vi "Main.vi"(8 "error in":errorcluster, 11 "Query Data in":refnum<class "Query Data.lvclass">) -> (0 "error out":errorcluster, 3 "Query Data out":refnum<class "Query Data.lvclass">)   [LabVIEW 2018, in "Query Data.lvclass"]
doc: "The Queued Message Handler of a Worker."
uses:
  Query Data.lvclass
  D:/Program Files (x86)/National Instruments/LabVIEW 2018/vi.lib/addons/_Workers/Library/Classes/Worker/Worker.lvclass
  Initialization Data.ctl
  Query Data.lvclass/Query Data.ctl
  <vilib>/drjdpowell/SQLite Library/SQL Connection/Open (path).vi
  <vilib>/drjdpowell/SQLite Library/SQL Connection/Open (string).vi
  <vilib>/AdvancedString/Path To Command Line String.vi
  <vilib>/drjdpowell/SQLite Library/SQL Connection/Execute SQL.vi
  <vilib>/addons/_Workers/Library/Classes/Message/Enqueue Message to Self v2.vi
  <vilib>/drjdpowell/SQLite Library/SQL Connection/Connection.lvclass
  <vilib>/addons/_Workers/Library/Classes/Worker/Worker.lvclass
  <vilib>/addons/_Workers/Library/Classes/Message/Message.lvclass
  <vilib>/drjdpowell/SQLite Library/SQLite.lvlib
  D:/Program Files (x86)/National Instruments/LabVIEW 2018/vi.lib/addons/_Workers/Library/Classes/Workers Object/Workers Object.lvclass
panel:
  in  "Query Button":bool
  in  "EndTime":timestamp caption="EndTime:"
  in  "StartTime":timestamp caption="StartTime:"
  in  "Slot":T1(ring) caption="Slot:"
  in  "Results":i32(listbox)
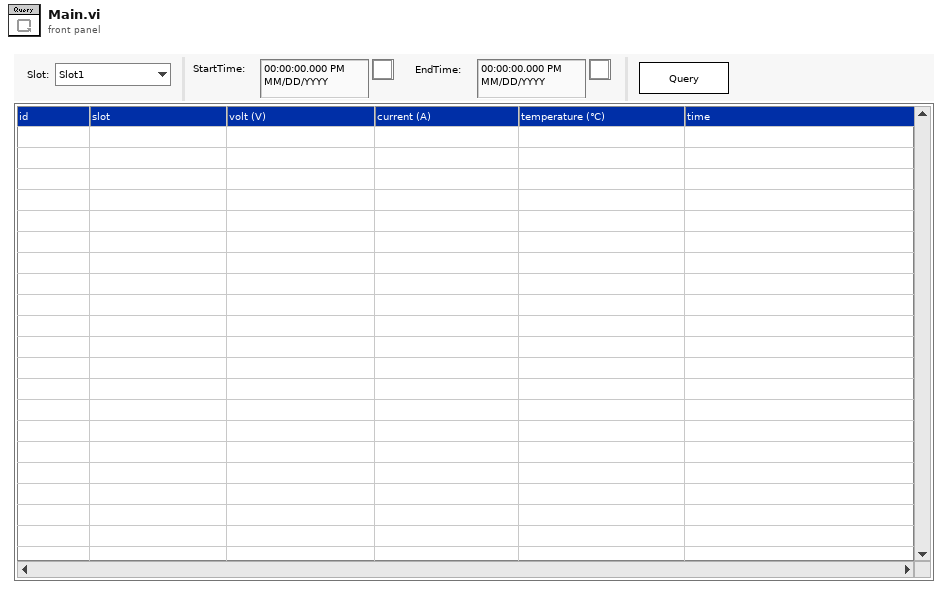
[diagram p1: front panel]
types:
  T1 = enum16{"Slot1", "Slot2", "Slot3", "Slot4", "Slot5", "Slot6", "Slot7", "Slot8", "Slot9", "Slot10"}
  T2 = typedef "Query Data.lvclass/Initialization Data.ctl" = cluster{"MainPanel":refnum<vi>}
  T3 = typedef "Workers.lvlib/Case Label.ctl" = string
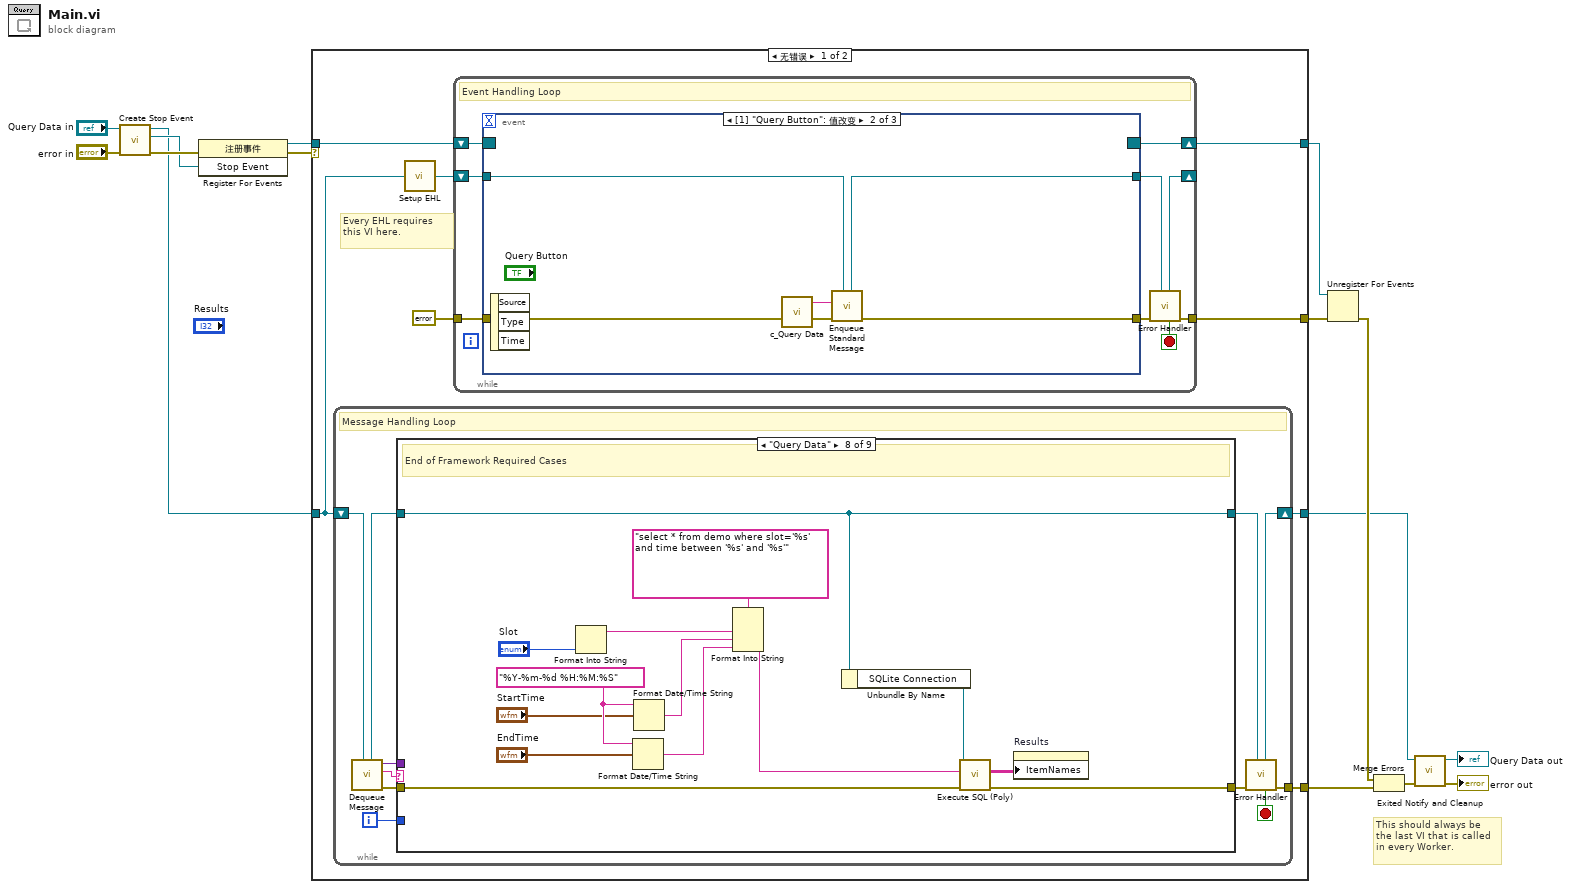
[diagram p0: block diagram]
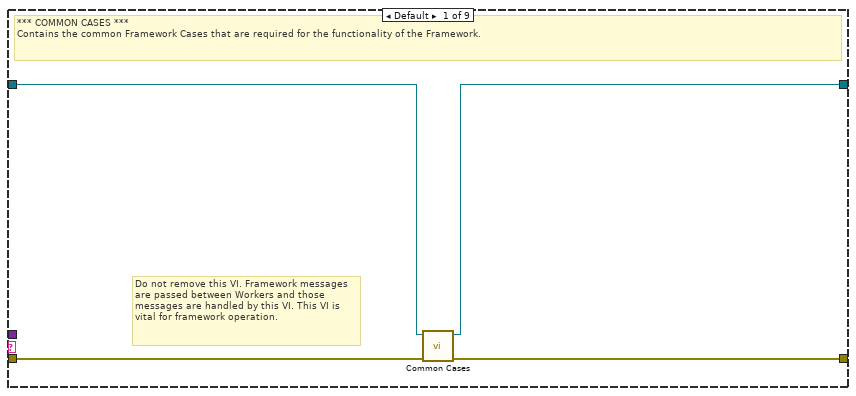
[diagram p2: hidden frame]
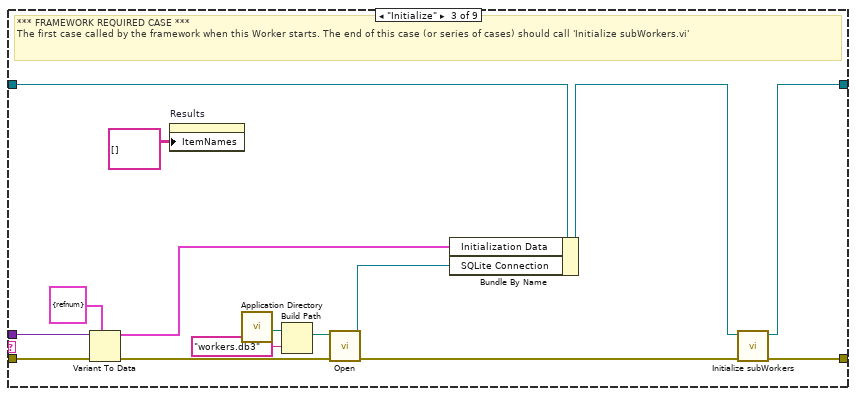
[diagram p4: hidden frame]
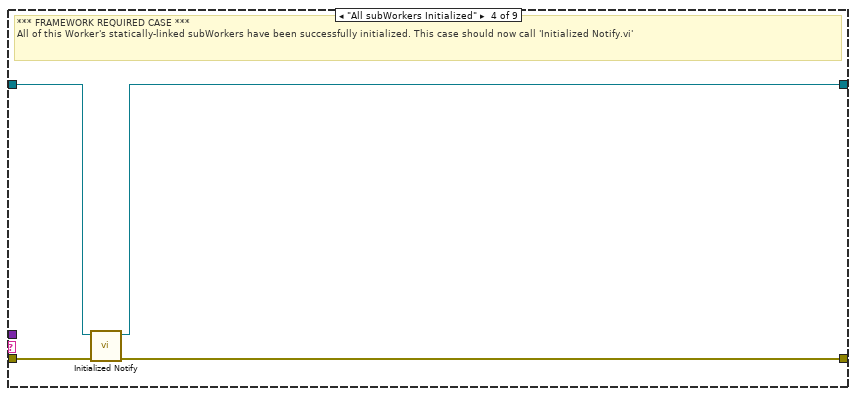
[diagram p5: hidden frame]
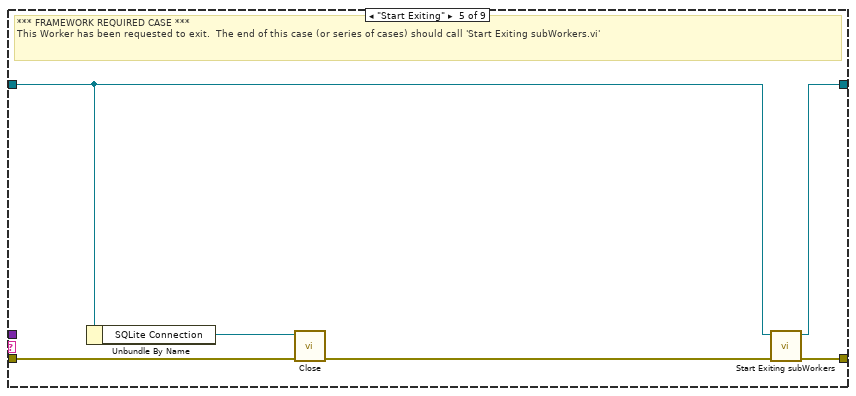
[diagram p6: hidden frame]
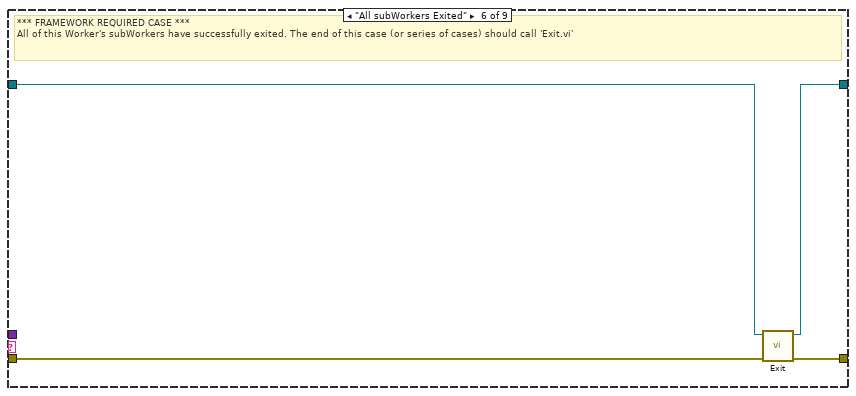
[diagram p7: hidden frame]
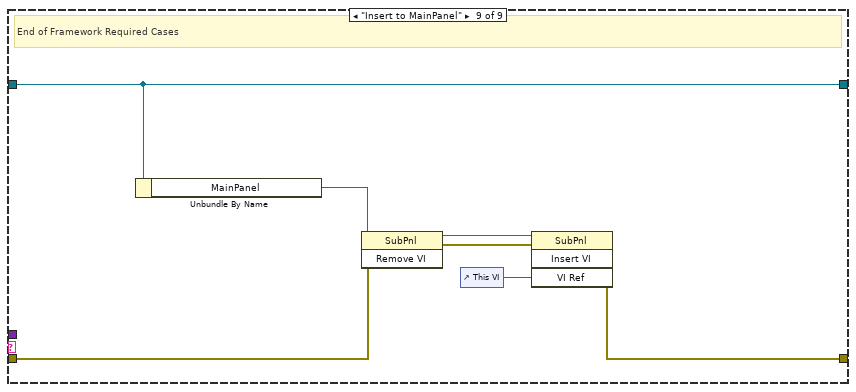
[diagram p9: hidden frame]
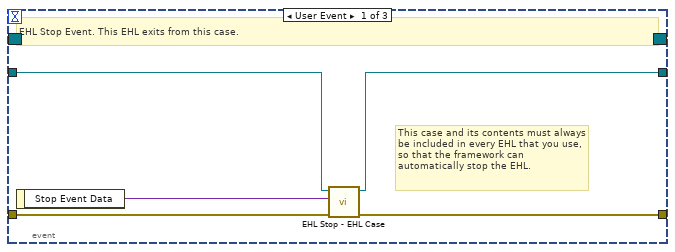
[diagram p10: hidden frame]
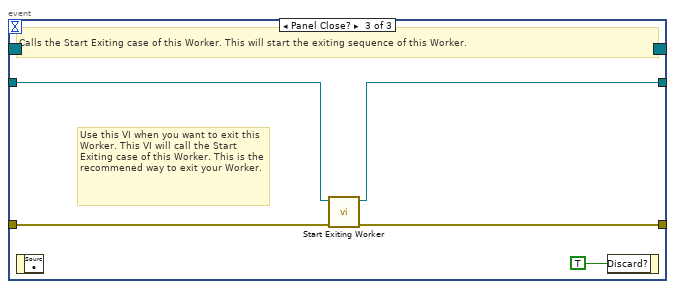
[diagram p11: hidden frame]
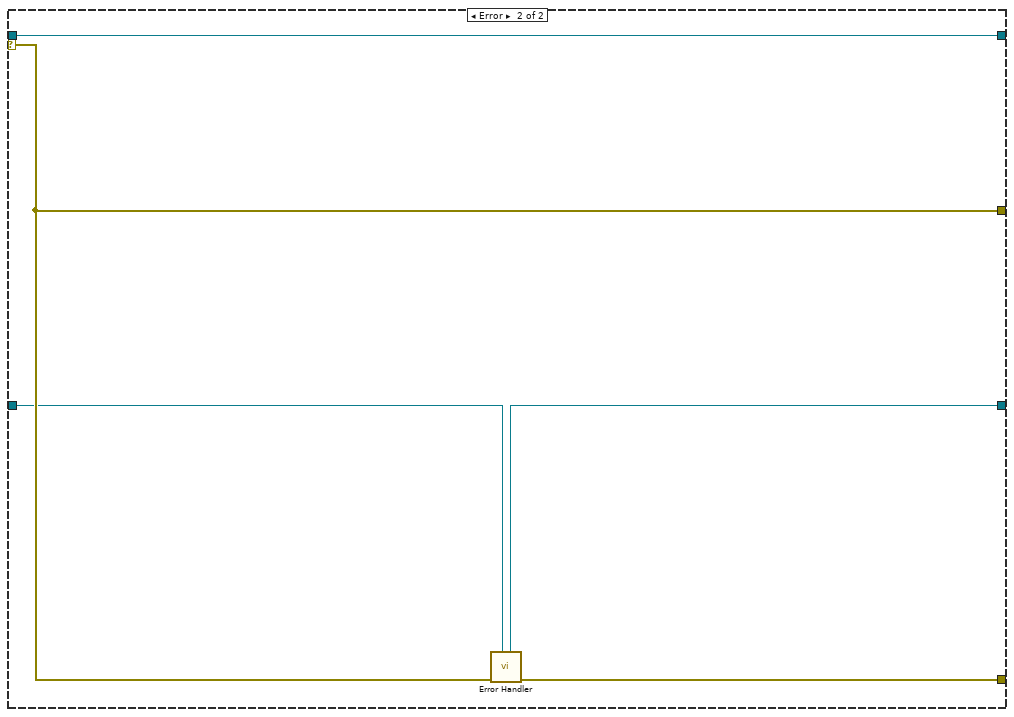
[diagram p12: hidden frame]
diagram:
  # "This should always be the last VI that is called in every Worker."
  n1 = call-dynamic "Create Stop Event.vi"("error in"="error in", "Worker"="Query Data in") -> ("error out"=w10:errorcluster, "Stop Event"=w7:refnum<user-event>, "Worker out"=w4:refnum<class "Query Data.lvclass">)  [unwired: 7 in]
  n2 = register-events(error in=w10, w7) -> (reference out=w9:refnum<event-registration>, error out=w1:errorcluster)  [unwired: 1 in]
  n3 = case shown="无错误" w1 {
    tunnel: w4 -> [w18 w118]
    tunnel: [w16 w119] -> w8
    tunnel: w9 -> [w23 w120]
    tunnel: [w20 w121] -> w14
    tunnel: [w22 w120] -> w13
    tunnel: [w17 w117] -> w11
    selector: w1 -> [_ w121]
    frame No Error {
      # "Every EHL requires\nthis VI here."
      n4 = while {
        shift-right: [w32] -> w17
        shift-left: w18 -> [w34]
        tunnel: [w33] -> w16
        i -> [w24]
        stop <- w25 stop-if-true
        # "Message Handling Loop"
        n5 = call-dynamic "Dequeue Message.vi"("Worker"=w34) -> ("error out"=w31:errorcluster, "Case out"=w26:string, "Data out"=w27:variant, "Worker out"=w29:refnum<class "Query Data.lvclass">)  [unwired: 6 in, 1 out]
        n6 = case "Worker MHL Case Structure (DO NOT CHANGE LABEL NAME)" shown="\"Query Data\"" w26 {
          tunnel: w31 -> [w38 w39 w53 w57 w62 w69 w70 w84 w87]
          tunnel: [w37 w39 w55 w56 w65 w68 w70 w83 w86] -> w30
          tunnel: w29 -> [w36 w40 w52 w59 w63 w67 w71 w85 w88]
          tunnel: [w35 w40 w54 w58 w64 w66 w71 w85 w88] -> w28
          tunnel: w27 -> [_ _ w51 _ _ _ _ _ _]
          tunnel: w24 -> [_ _ _ _ _ _ _ _ _]
          frame Default {
            # "Do not remove this VI. Framework messages are passed between Workers and those messages are handled by this VI. This VI is vital for framework operation."
            # "*** COMMON CASES ***\nContains the common Framework Cases that are required for the functionality of the Framework."
            n7 = call-dynamic "Common Cases.vi"("error in"=w38, "Worker in"=w36) -> ("error out"=w37:errorcluster, "Worker out"=w35:refnum<class "Query Data.lvclass">)  [unwired: 8 in]
          }
          frame "------ FRAMEWORK REQUIRED CASES ------" {
            # "Start of Framework Required Cases"
          }
          frame "Initialize" {
            # "*** FRAMEWORK REQUIRED CASE ***\nThe first case called by the framework when this Worker starts. The end of this case (or series of cases) should call 'Initialize subWorkers.vi'"
            n8 = Variant To Data(error in=w53, type=T2 {"MainPanel"=refnum} ("Initialization Data"), Variant=w51) -> (data=w48:T2, error out=w47:errorcluster)
            n9 = property on="Results" class="MCListbox (严格)"("ItemNames"=string[][] [] ("Item Names")) -> ()  [unwired: 2 in, 2 out]
            n10 = call <vilib>:"Application Directory.vi"() -> ("Application Directory"=w46:path)
            n11 = Build Path(base path=w46, name or relative path="workers.db3") -> (appended path=w44:path)
            n12 = call-poly <vilib>:"Open.vi"("error in (no error)"=w47, "db file"=w44) -> ("error out"=w42:errorcluster, "SQLite Connection"=w43:refnum<class "Connection.lvclass">)  [unwired: 8 in]
            n13 = Bundle By Name(cluster=w52, "Initialization Data"=w48, "SQLite Connection"=w43) -> (w49:refnum<class "Query Data.lvclass">)
            n14 = call-dynamic "Initialize subWorkers.vi"("error in"=w42, "Worker"=w49) -> ("error out"=w55:errorcluster, "dup Worker out"=w54:refnum<class "Query Data.lvclass">)  [unwired: 8 in]
          }
          frame "All subWorkers Initialized" {
            # "*** FRAMEWORK REQUIRED CASE ***\nAll of this Worker's statically-linked subWorkers have been successfully initialized. This case should now call 'Initialized Notify.vi'"
            n15 = call-dynamic "Initialized Notify.vi"("error in"=w57, "Worker"=w59) -> ("error out"=w56:errorcluster, "dup Worker out"=w58:refnum<class "Query Data.lvclass">)  [unwired: 8 in]
          }
          frame "Start Exiting" {
            # "*** FRAMEWORK REQUIRED CASE ***\nThis Worker has been requested to exit.  The end of this case (or series of cases) should call 'Start Exiting subWorkers.vi'"
            n16 = Unbundle By Name(w63) -> ("SQLite Connection"=w60:refnum<class "Connection.lvclass">)
            n17 = call-dynamic "Close.vi"("error in (no error)"=w62, "SQLite Connection in"=w60) -> ("error out"=w61:errorcluster)  [unwired: 9 in]
            n18 = call-dynamic "Start Exiting subWorkers.vi"("error_in"=w61, "Worker"=w63) -> ("error out"=w65:errorcluster, "dup Worker out"=w64:refnum<class "Query Data.lvclass">)  [unwired: 8 in]
          }
          frame "All subWorkers Exited" {
            # "*** FRAMEWORK REQUIRED CASE ***\nAll of this Worker's subWorkers have successfully exited. The end of this case (or series of cases) should call 'Exit.vi'"
            n19 = call-dynamic "Exit.vi"("error_in"=w69, "Worker"=w67) -> ("error out"=w68:errorcluster, "dup Worker out"=w66:refnum<class "Query Data.lvclass">)  [unwired: 8 in]
          }
          frame "-----------------------------------------------" {
            # "End of Framework Required Cases"
          }
          frame "Query Data" {
            w80 = "%Y-%m-%d %H:%M:%S" ("time format string (%c)")
            # "End of Framework Required Cases"
            n20 = Format Into String("Slot") -> (resulting string=w76:string)  [unwired: 3 in, 1 out]
            n21 = Format Date/Time String(time format string (%c)=w80, seconds (now)="EndTime") -> (date/time string=w74:string)  [unwired: 1 in]
            n22 = Format Date/Time String(time format string (%c)=w80, seconds (now)="StartTime") -> (date/time string=w75:string)  [unwired: 1 in]
            n23 = Format Into String(format string="select * from demo where slot='%s' and time between '%s' and '%s'", w76, w75, w74) -> (resulting string=w73:string)  [unwired: 2 in, 1 out]
            n24 = Unbundle By Name(w85) -> ("SQLite Connection"=w82:refnum<class "Connection.lvclass">)
            n25 = call-poly <vilib>:"Execute SQL (Poly).vi"("error in (no error)"=w84, "SQL"=w73, "SQLite Connection in"=w82) -> ("error out"=w83:errorcluster, "Result Set"=w72:string[][])  [unwired: 5 in, 2 out]
            n26 = property on="Results" class="MCListbox (严格)"("ItemNames"=w72) -> ()  [unwired: 2 in, 2 out]
          }
          frame "Insert to MainPanel" {
            # "End of Framework Required Cases"
            n27 = Unbundle By Name(w88) -> ("MainPanel"=w92:refnum<vi>)
            n28 = invoke class="SubPnl" method="Remove VI"(reference=w92, error in=w87) -> (reference out=w91:refnum<vi>, error out=w90:errorcluster)  [unwired: 1 in, 1 out]
            n29 = control-ref of="This VI"() -> (w89:refnum<vi>)
            n30 = invoke class="SubPnl" method="Insert VI"(reference=w91, error in=w90, "VI Ref"=w89) -> (error out=w86:errorcluster)  [unwired: 1 in, 3 out]
          }
        }
        n31 = call-dynamic "Error Handler.vi"("Worker"=w28, "error_in"=w30) -> ("error out"=w33:errorcluster, "Stop Loop"=w25:bool, "Worker out"=w32:refnum<class "Query Data.lvclass">)  [unwired: 7 in]
      }
      n32 = call-dynamic "Setup EHL.vi"("Worker"=w18) -> ("Worker out"=w19:refnum<class "Query Data.lvclass">)  [unwired: 14 in]
      n33 = while "Event Handling Loop" {
        shift-right: [w101] -> w22
        shift-left: w23 -> [w100]
        tunnel: [w96] -> w20
        tunnel: errorcluster {"status"=FALSE, "code"=0, "source"=""} ("error constant") -> [w98]
        shift-right: [w94] -> _
        shift-left: w19 -> [w99]
        stop <- w93 stop-if-true
        # "Event Handling Loop"
        n34 = event shown="[1] \"Query Button\": 值改变" {
          selector: w100 -> [_ _ _]
          dyn-events: [_ _ _] -> w101
          timeout: _ -> [_ _ _]
          tunnel: [w105 w110 w115] -> w97
          tunnel: w98 -> [w106 w111 w114]
          tunnel: w99 -> [w104 w109 w113]
          tunnel: [w103 w108 w112] -> w95
          event User Event {
            # "This case and its contents must always be included in every EHL that you use, so that the framework can automatically stop the EHL."
            # "EHL Stop Event. This EHL exits from this case."
            n35 = event-data() -> ("Stop Event Data"=w102:variant)  [unwired: 1 in]
            n36 = call <vilib>:"EHL Stop - EHL Case.vi"("error in"=w106, "Stop Event Data"=w102, "Worker"=w104) -> ("error out"=w105:errorcluster, "Worker out"=w103:refnum<class "Query Data.lvclass">)  [unwired: 7 in]
          }
          event "Query Button": Value Change {
            n37 = event-data() -> ()  [unwired: 1 in, 3 out]
            n38 = call "c_Query Data.vi"() -> ("Case Label"=w107:T3)  [unwired: 1 in]
            n39 = call-poly <vilib>:"Enqueue Standard Message.vi"("Worker"=w109, "error in"=w111, "Case Label"=w107) -> ("error out"=w110:errorcluster, "dup Worker out"=w108:refnum<class "Query Data.lvclass">)  [unwired: 7 in]
          }
          event Panel Close? {
            # "Use this VI when you want to exit this Worker. This VI will call the Start Exiting case of this Worker. This is the recommened way to exit your Worker."
            # "Calls the Start Exiting case of this Worker. This will start the exiting sequence of this Worker."
            n40 = event-data() -> ()  [unwired: 1 in, 1 out]
            n41 = call-dynamic "Start Exiting Worker.vi"("error in"=w114, "Worker"=w113) -> ("error out"=w115:errorcluster, "dup Worker out"=w112:refnum<class "Query Data.lvclass">)  [unwired: 8 in]
            n42 = event-data("Discard?"=TRUE) -> ()  [unwired: 1 in, 1 out]
          }
        }
        n43 = call-dynamic "Error Handler.vi"("Worker"=w95, "error_in"=w97) -> ("error out"=w96:errorcluster, "Stop Loop"=w93:bool, "Worker out"=w94:refnum<class "Query Data.lvclass">)  [unwired: 7 in]
      }
    }
    frame Error {
      n44 = call-dynamic "Error Handler.vi"("Worker"=w118, "error_in"=w121) -> ("error out"=w119:errorcluster, "Worker out"=w117:refnum<class "Query Data.lvclass">)  [unwired: 7 in, 1 out]
    }
  }
  n45 = Unregister For Events(event registration refnum=w13, error in=w14) -> (error out=w15:errorcluster)
  n46 = Merge Errors(w15, w8) -> (w12:errorcluster)
  n47 = call-dynamic "Exited Notify and Cleanup.vi"("error_in"=w12, "Worker"=w11) -> ("error out"=→"error out":errorcluster, "dup Worker out"=→"Query Data out":refnum<class "Query Data.lvclass">)  [unwired: 8 in]
